vi "GetMessageDataType.vi"(8 "error in":errorcluster, 11 "message":T2) -> (0 "error out":errorcluster, 3 "data type":T1)   [LabVIEW 2013, in "CLM_LocalMessage.lvclass"]
uses:
  CLM_LocalMessage.lvclass
  Message.ctl
  <vilib>/Utility/VariantDataType/Type.ctl
  <vilib>/Utility/VariantDataType/VariantType.lvlib
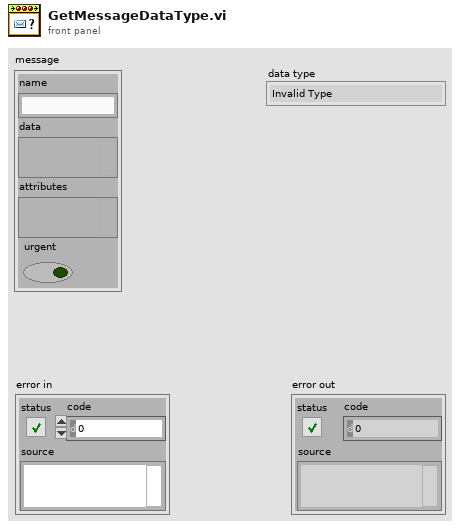
[diagram p1: front panel]
types:
  T1 = typedef "VariantType.lvlib/Type.ctl" = enum8{"Invalid Type", "Void", "I8", "I16", "I32", "I64", "U8", "U16", "U32", "U64", "Single Float", "Double Float", "Extended Float", "Single Complex", "Double Complex", "Extended Complex", "Enum U8", "Enum U16", "Enum U32", "Enum U64", "Single Float With Unit", "Double Float With Unit", "Extended Float With Unit", "Single Complex with Unit", "Double Complex with Unit", "Extended Complex with Unit", "Boolean", "String", "Path", "Picture", "Tag", "Array", "Cluster", "Variant", "LV Variant", "Waveform", "Timestamp", "Digital Waveform", "Digital Data", "ExpressData", "Refnum", "External Data", "VI", "Poly VI", "LabVIEW Class Instance", "Fixed Point"}
  T2 = typedef "CLM_LocalMessage.lvclass/Message.ctl" = cluster{"name":string, "data":variant, "attributes":variant, "urgent":bool}
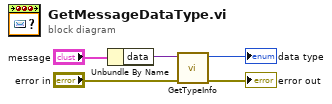
[diagram p0: block diagram]
diagram:
  n1 = Unbundle By Name("message") -> ("data"=w4:variant)
  n2 = call <vilib>:"GetTypeInfo.vi"("error in (no error)"="error in", "Variant"=w4) -> ("error out"=→"error out":errorcluster, "Type Enum"=→"data type":T1)  [unwired: 5 in, 3 out]
